vi "StationCmdsGlobal.vi"() -> ()   [LabVIEW 2016]
uses:
  StationCmds.ctl
  ZAddress.ctl
  Scope_Model.ctl
panel:
  out "PW(T)/CW(F)":bool
  in  "Mode_selection":enum32{"PW-mode", "CW-mode"}(radio)
  in  "USB Address":refnum<visa-resource-name>="USB0::0x05FF::0x1023::3511N16147::INSTR"
  in  "LeCroy Model":T1=3 items=["9400", "9420 / 9450", "9310", "LT342,262", "S 432", "HDO4034"]
  out "next cell top-right":cluster{"row":i32, "column":i32}
  in  "Print Data?":bool
  in  "Quit":bool
  in  "HydrophoneID":i32=4085
  in  "Z Address":T2={"Address"="192.168.52.121", "Port"=1023}
  in  "StationCmds":T3={"scopeSn"="2", "imagingHwConfig"="1", "scopeSampleNum"=1000, "scopeSampleInc"=1e-08, "zStartDistCm"=3.0, "zMeasNum"=0, "zIncrementCm"=0.0, "profRangeLimitDb"=15.0, "profMinNum"=9, "profIncrementCm"=0.025, "siiZLimitDb"=0.0, "siiZMinNum"=0, "siiZIncrementCm"=0.0, "Hydro sens (dB)"=-270.0} {"siiZIncrementCm" format="%.2f"; "siiZLimitDb" format="%.2f"; "profIncrementCm" format="%.2f"; "profRangeLimitDb" format="%.2f"; "zIncrementCm" format="%.2f"; "Hydro sens (dB)" format="%.2f"; "scopeSampleInc" format="%.2e"; "zStartDistCm" format="%.2f"}
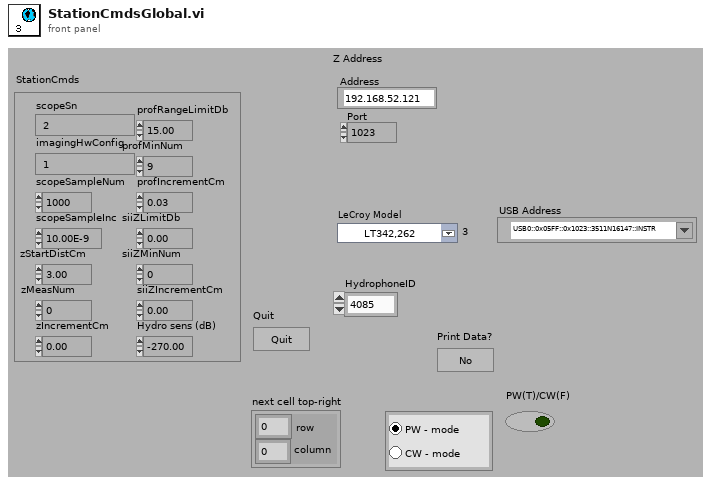
[diagram p1: front panel]
types:
  T1 = typedef "Scope_Model.ctl" = u16
  T2 = typedef "ZAddress.ctl" = cluster{"Address":string, "Port":u16}
  T3 = typedef "StationCmds.ctl" = cluster{"scopeSn":string, "imagingHwConfig":string, "scopeSampleNum":i16, "scopeSampleInc":sgl, "zStartDistCm":sgl, "zMeasNum":i16, "zIncrementCm":sgl, "profRangeLimitDb":sgl, "profMinNum":i8, "profIncrementCm":sgl, "siiZLimitDb":sgl, "siiZMinNum":i8, "siiZIncrementCm":sgl, "Hydro sens (dB)":sgl}
diagram:
